vi "Delete Attribute Tree Data.vi"(7 "Tree ID":string, 8 "Error In":errorcluster, 10 "Attribute Name":string, 11 "Tree Manager":refnum<data-value>) -> (0 "Error Out":errorcluster, 1 "Attribute Value":refnum<class "Tree Data.lvclass">, 2 "Found?":bool, 3 "Tree Manager":refnum<data-value>)   [LabVIEW 2017, in "Tree API.lvlib" / "Tree.lvclass"]
doc: "Delete a Tree Data typed attribute from the Tree and return it."
uses:
  Tree.lvclass
  Tree Data/Tree Data.lvclass
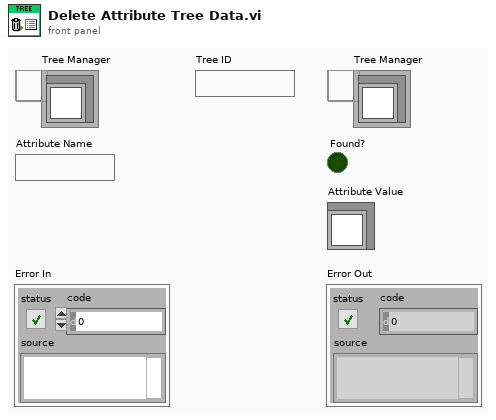
[diagram p1: front panel]
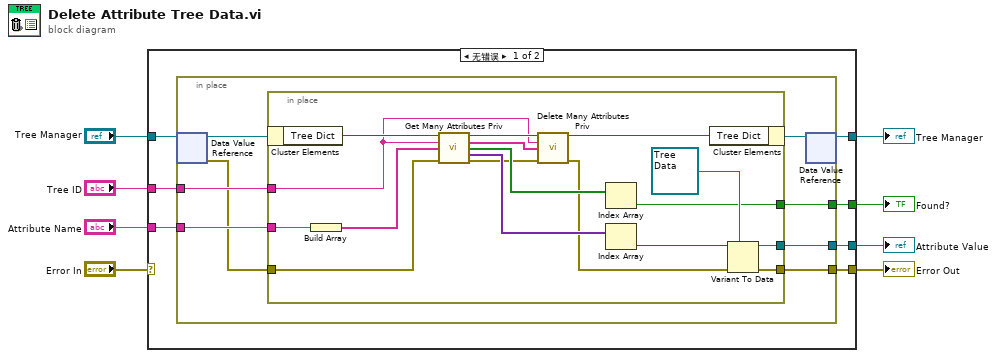
[diagram p0: block diagram]
diagram:
  n1 = case shown="无错误" "Error In" {
    selector: "Error In" -> [_ w41]
    tunnel: "Tree Manager" -> [w15 w42]
    tunnel: [w14 w42] -> w7
    tunnel: [w13 w41] -> w5
    tunnel: "Tree ID" -> [w12 _]
    tunnel: "Attribute Name" -> [w11 _]
    tunnel: [w10 _] -> w2
    tunnel: [w9 _] -> w1
    frame No Error {
      n2 = in-place {
        in-place-border: [w19] -> w13
        in-place-border: w12 -> [w22]
        in-place-border: w11 -> [w21]
        in-place-border: [w17] -> w10
        in-place-border: [w18] -> w9
        n3 = in-place-dvr #1(w15) -> (w23:refnum<class "Tree.lvclass">, w20:errorcluster)
        n4 = in-place {
          in-place-border: [w40] -> w19
          in-place-border: w20 -> [w34]
          in-place-border: w22 -> [w27]
          in-place-border: w21 -> [w36]
          in-place-border: [w32] -> w17
          in-place-border: [w38] -> w18
          n5 = in-place-cluster #2(w23) -> ("Tree Dict"=w37:variant)
          n6 = Build Array(w36) -> (w35:string[])
          n7 = call "Get Many Attributes Priv.vi"("Tree Dictionary In"=w37, "Unique ID"=w27, "Attribute Names"=w35, "error in"=w34) -> ("Tree Dictionary Out"=w29:variant, "Attribute Names"=w28:string[], "Found?"=w33:bool[], "Attribute Values"=w31:variant[], "error out"=w24:errorcluster)  [unwired: 6 in, 1 out]
          n8 = call "Delete Many Attributes Priv.vi"("Tree Dictionary In"=w29, "Unique ID"=w27, "Attribute Names"=w28, "error in"=w24) -> ("Tree Dictionary Out"=w26:variant, "error out"=w25:errorcluster)  [unwired: 10 in]
          n9 = Index Array(array=w33) -> (element=w32:bool)  [unwired: 1 in]
          n10 = Index Array(array=w31) -> (element=w30:variant)  [unwired: 1 in]
          n11 = in-place-cluster #2("Tree Dict"=w26) -> (w16:refnum<class "Tree.lvclass">)
          n12 = Variant To Data(error in=w25, type=refnum<class "Tree Data.lvclass"> refnum ("Tree Data.lvclass"), Variant=w30) -> (data=w38:refnum<class "Tree Data.lvclass">, error out=w40:errorcluster)
        }
        n13 = in-place-dvr #1(w16) -> (w14:refnum<data-value>)  [unwired: 1 out]
      }
    }
    frame Error {
    }
  }
  "Tree Manager" <- w7
  "Error Out" <- w5
  "Found?" <- w2
  "Attribute Value" <- w1
